vi "Finish.vi"   [LabVIEW 2012]
doc: "This VI is called just before exiting. It is expected to close I/O refnum, save collected data, etc."
uses:
  <vilib>/Rock Robotics/WPI/Compressor/WPI_CompressorGetSetRefNum.vi
  <vilib>/Rock Robotics/WPI/RobotDrive/WPI_RobotDriveGetSetRefNum.vi
  <vilib>/Rock Robotics/WPI/Joystick/WPI_JoystickGetSetRefNum.vi
types:
  T1 = typedef "WPI_CameraDevRef.ctl" = cluster{"Camera Address":string, "CameraStatus":errorcluster, "Acquire Image Notifier":refnum<notifier>}
  T2 = typedef "WPI_JoystickDevRef.ctl" = cluster{"Device":T3}
  T3 = typedef "WPI_JoystickDeviceEnum.ctl" = enum16{"USB 1", "USB 2", "USB 3", "USB 4", "Kinect 1", "Kinect 2"}
  T4 = typedef "WPI_RobotDriveDevRef.ctl" = cluster{"DevStatus":errorcluster, "Motors[]":T5[], "Square Inputs":bool, "Max Output":dbl, "Isochronous":bool}
  T5 = typedef "WPI_MotorControlDeviceRef.ctl" = cluster{"DeviceStatus":errorcluster, "Type":enum16{"PWM", "CAN"}, "PWM":cluster{"Digital Module":T6, "PWM Channel":T7, "DeadBand":T8}, "CAN":cluster{"Device Number":u8, "Control Mode":T9, "Semaphore":T10, "Max Vout":dbl}, "Invert":bool, "TransformRef":T11, "InvTransformRef":T11}
  T6 = typedef "FPGA_TypedefDigitalModule.ctl" = enum16{"Digital Module 1", "Digital Module 2"}
  T7 = typedef "FPGA_DIOPWMChannel.ctl" = enum8{"PWM 1", "PWM 2", "PWM 3", "PWM 4", "PWM 5", "PWM 6", "PWM 7", "PWM 8", "PWM 9", "PWM 10", "Invalid"}
  T8 = typedef "WPI_PWMDeadband.ctl" = cluster{"Name":string, "maxPositivePwm":i32, "minPositivePwm":i32, "centerPwm":i32, "maxNegativePwm":i32, "minNegativePwm":i32, "angularRange":u16}
  T9 = typedef "WPI_CANJaguar_ControlMode.ctl" = enum8{"Percent VBus", "Current", "Speed", "Position", "Voltage"}
  T10 = typedef "Semaphore RefNum" = refnum<k1>
  T11 = typedef "WPI_PWMTransform_ConPane.ctl" = refnum<vi>
  T12 = typedef "WPI_SolenoidDevRef.ctl" = cluster{"DevStatus":errorcluster, "Solenoid Module":T13, "Forward Solenoid Channel":T14, "Reverse Solenoid Channel":T14}
  T13 = typedef "FPGA_TypedefSolenoidModule.ctl" = enum16{"Solenoid Module 1", "Solenoid Module 2"}
  T14 = typedef "WPI_SolenoidChannel.ctl" = enum8{"Solenoid 1", "Solenoid 2", "Solenoid 3", "Solenoid 4", "Solenoid 5", "Solenoid 6", "Solenoid 7", "Solenoid 8", "Invalid"}
  T15 = typedef "WPI_CompressorDevRef.ctl" = cluster{"DevStatus":errorcluster, "DigitalInputDevRef":T16, "RelayDevRef":T18}
  T16 = typedef "WPI_DigitalInputDevRef.ctl" = cluster{"DevStatus":errorcluster, "DIO Channel":T17, "Digital Module":T6}
  T17 = typedef "FPGA_DIOChannel.ctl" = enum8{"DIO 1", "DIO 2", "DIO 3", "DIO 4", "DIO 5", "DIO 6", "DIO 7", "DIO 8", "DIO 9", "DIO 10", "DIO 11", "DIO 12", "DIO 13", "DIO 14", "Invalid"}
  T18 = typedef "WPI_RelayDevRef.ctl" = cluster{"DevStatus":errorcluster, "Relay Channel":T19, "Digital Module":T6, "Relay Direction":T20}
  T19 = typedef "FPGA_DIORelayChannel.ctl" = enum8{"Relay 1", "Relay 2", "Relay 3", "Relay 4", "Relay 5", "Relay 6", "Relay 7", "Relay 8", "Invalid"}
  T20 = typedef "WPI_RelayDirection.ctl" = enum16{"Both directions", "Forward only", "Reverse only"}
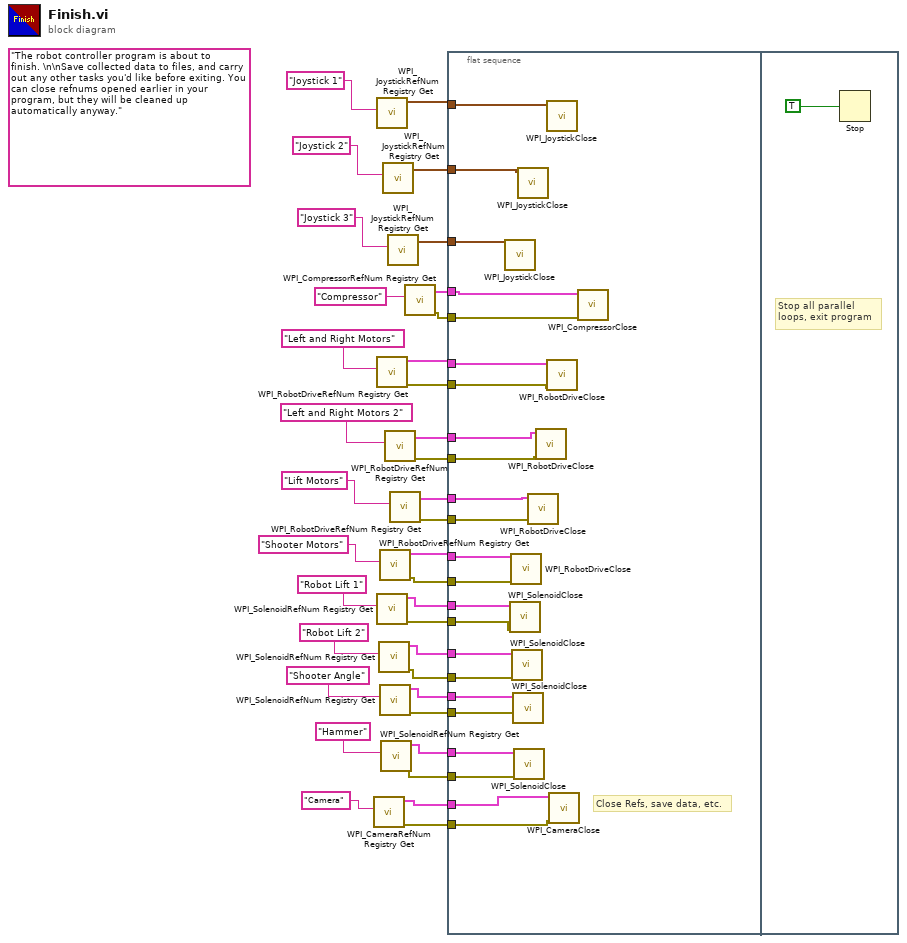
[diagram p0: block diagram]
diagram:
  (unwired) "The robot controller program is about to finish. \n\nSave collected data to files, and carry out any other tasks you'd like before exiting. You can close refnums opened earlier in your program, but they will be cleaned up automatically anyway."
  n1 = call <vilib>:"WPI_CameraRefNum Registry Get.vi"("refnum name"="Camera") -> ("error out"=w10:errorcluster, "CameraDevRef"=w32:T1)  [unwired: 1 in, 8 out]
  n2 = call <vilib>:"WPI_JoystickRefNum Registry Get.vi"("refnum name"="Joystick 1") -> ("JoystickDevRef"=w33:T2)  [unwired: 1 in, 9 out]
  n3 = call <vilib>:"WPI_RobotDriveRefNum Registry Get.vi"("refnum name"="Left and Right Motors") -> ("error out"=w2:errorcluster, "RobotDriveDevRef"=w34:T4)  [unwired: 1 in, 8 out]
  n4 = call <vilib>:"WPI_SolenoidRefNum Registry Get.vi"("refnum name"="Robot Lift 1") -> ("error out"=w6:errorcluster, "SolenoidDevRef"=w18:T12)  [unwired: 9 in]
  n5 = call <vilib>:"WPI_SolenoidRefNum Registry Get.vi"("refnum name"="Robot Lift 2") -> ("error out"=w7:errorcluster, "SolenoidDevRef"=w16:T12)  [unwired: 9 in]
  n6 = call <vilib>:"WPI_RobotDriveRefNum Registry Get.vi"("refnum name"="Shooter Motors") -> ("error out"=w5:errorcluster, "RobotDriveDevRef"=w21:T4)  [unwired: 9 in]
  n7 = call <vilib>:"WPI_SolenoidRefNum Registry Get.vi"("refnum name"="Shooter Angle") -> ("error out"=w8:errorcluster, "SolenoidDevRef"=w15:T12)  [unwired: 9 in]
  n8 = call <vilib>:"WPI_SolenoidRefNum Registry Get.vi"("refnum name"="Hammer") -> ("error out"=w9:errorcluster, "SolenoidDevRef"=w14:T12)  [unwired: 9 in]
  n9 = call <vilib>:"WPI_JoystickRefNum Registry Get.vi"("refnum name"="Joystick 2") -> ("JoystickDevRef"=w29:T2)  [unwired: 1 in, 9 out]
  n10 = call <vilib>:"WPI_RobotDriveRefNum Registry Get.vi"("refnum name"="Left and Right Motors 2") -> ("error out"=w3:errorcluster, "RobotDriveDevRef"=w27:T4)  [unwired: 1 in, 8 out]
  n11 = call <vilib>:"WPI_JoystickRefNum Registry Get.vi"("refnum name"="Joystick 3") -> ("JoystickDevRef"=w23:T2)  [unwired: 1 in, 9 out]
  n12 = call <vilib>:"WPI_RobotDriveRefNum Registry Get.vi"("refnum name"="Lift Motors") -> ("error out"=w4:errorcluster, "RobotDriveDevRef"=w25:T4)  [unwired: 9 in]
  n13 = call <vilib>:"WPI_CompressorRefNum Registry Get.vi"("refnum name"="Compressor") -> ("error out"=w1:errorcluster, "CompressorDevRef"=w19:T15)  [unwired: 9 in]
  n14 = flat-sequence {
    tunnel: w34 -> [w59]
    tunnel: w33 -> [w58]
    tunnel: w32 -> [w57]
    tunnel: w29 -> [w56]
    tunnel: w27 -> [w55]
    tunnel: w25 -> [w54]
    tunnel: w23 -> [w53]
    tunnel: w21 -> [w52]
    tunnel: w19 -> [w51]
    tunnel: w18 -> [w50]
    tunnel: w16 -> [w49]
    tunnel: w15 -> [w48]
    tunnel: w14 -> [w47]
    tunnel: w10 -> [w46]
    tunnel: w9 -> [w45]
    tunnel: w8 -> [w44]
    tunnel: w7 -> [w43]
    tunnel: w6 -> [w42]
    tunnel: w5 -> [w41]
    tunnel: w4 -> [w40]
    tunnel: w3 -> [w39]
    tunnel: w2 -> [w38]
    tunnel: w1 -> [w37]
    frame #0 {
      # "Close Refs, save data, etc."
      n15 = call <vilib>:"WPI_JoystickClose.vi"("JoystickDevRef"=w53) -> ()  [unwired: 11 out]
      n16 = call <vilib>:"WPI_SolenoidClose.vi"("error in (no error)"=w42, "SolenoidDevRef"=w50) -> ()  [unwired: 9 in, 1 out]
      n17 = call <vilib>:"WPI_RobotDriveClose.vi"("error in (no error)"=w41, "RobotDriveDevRef"=w52) -> ()  [unwired: 10 out]
      n18 = call <vilib>:"WPI_SolenoidClose.vi"("error in (no error)"=w43, "SolenoidDevRef"=w49) -> ()  [unwired: 9 in, 1 out]
      n19 = call <vilib>:"WPI_SolenoidClose.vi"("error in (no error)"=w44, "SolenoidDevRef"=w48) -> ()  [unwired: 9 in, 1 out]
      n20 = call <vilib>:"WPI_SolenoidClose.vi"("error in (no error)"=w45, "SolenoidDevRef"=w47) -> ()  [unwired: 9 in, 1 out]
      n21 = call <vilib>:"WPI_JoystickClose.vi"("JoystickDevRef"=w56) -> ()  [unwired: 11 out]
      n22 = call <vilib>:"WPI_RobotDriveClose.vi"("error in (no error)"=w40, "RobotDriveDevRef"=w54) -> ()  [unwired: 10 out]
      n23 = call <vilib>:"WPI_RobotDriveClose.vi"("error in (no error)"=w39, "RobotDriveDevRef"=w55) -> ()  [unwired: 10 out]
      n24 = call <vilib>:"WPI_JoystickClose.vi"("JoystickDevRef"=w58) -> ()  [unwired: 11 out]
      n25 = call <vilib>:"WPI_RobotDriveClose.vi"("error in (no error)"=w38, "RobotDriveDevRef"=w59) -> ()  [unwired: 10 out]
      n26 = call <vilib>:"WPI_CameraClose.vi"("error in (no error)"=w46, "CameraDevRef"=w57) -> ()  [unwired: 10 out]
      n27 = call <vilib>:"WPI_CompressorClose.vi"("error in (no error)"=w37, "CompressorDevRef"=w51) -> ()  [unwired: 9 in, 1 out]
    }
    frame #1 {
      # "Stop all parallel\nloops, exit program"
      n28 = Stop(stop? (T)=TRUE ("Quit")) -> ()
    }
  }
